vi "MEScope_GetFirmwareVer.vi"(8 "error in (no error)":errorcluster) -> (0 "error out":errorcluster, 1 "return type":i32, 3 "pnFwVersion":i32)   [LabVIEW 2015]
doc: "MEScope_GetFirmwareVer\n\nDescription:\nThis test will return the version number of the firmware running in the Cypress.\nDetail:\nint MEScope_GetFirmwareVer (\nint * pnFwVersion\n);\nParameters:\nint * pnFwVersion- Pointer to a integer buffer, filled with the version number data.\n\nReturn Values:\nA returned value of 0 indicates success, with the appropriate strings in the buffer. Otherwise, treat the returned value as an error code."
uses:
  ScannerDiagDLL.dll
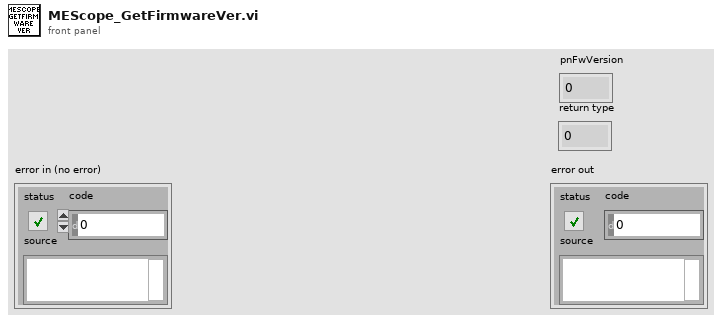
[diagram p1: front panel]
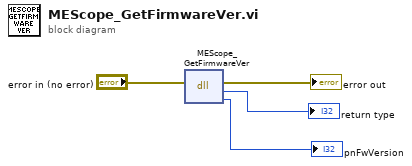
[diagram p0: block diagram]
diagram:
  n1 = dll-call lib="C:/ModisEdge/Scope/Test Sequence/Code Modules/DLL/ScannerDiagDLL.dll" fn="MEScope_GetFirmwareVer"(error in="error in (no error)") -> (error out=→"error out":errorcluster, "return type"=→"return type":i32, "pnFwVersion"=→"pnFwVersion":i32)  [unwired: 3 in, 1 out]
